vi "AlliGator Get HDF5 File Type.vi"(8 "Error In":errorcluster, 11 "File Path":path) -> (0 "Error Out":errorcluster, 3 "File Type":string)   [LabVIEW 2021, in "AlliGator HDF5.lvlib"]
uses:
  AlliGator HDF5.lvlib
  <vilib>/addons/h5labview2/base/hid_t.ctl
  <vilib>/addons/h5labview2/base/H5Equery.vi
  <vilib>/addons/h5labview2/base/lib_path.vi
  <vilib>/addons/h5labview2/dataset/H5Dread.llb/H5Dread.xnode
  <vilib>/addons/h5labview2/group/H5G.lvlib
  <vilib>/addons/h5labview2/file/H5F.lvlib
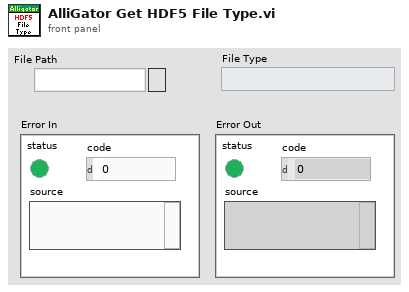
[diagram p1: front panel]
types:
  T1 = typedef "hid_t.ctl" = i64
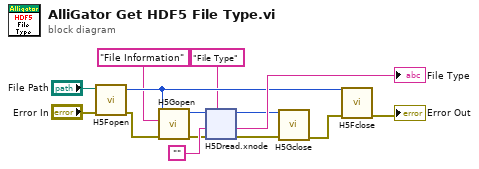
[diagram p0: block diagram]
diagram:
  n1 = call <vilib>:"H5Fopen.vi"("error in (no error)"="Error In", "path"="File Path") -> ("error out"=w3:errorcluster, "ref out"=w12:T1)  [unwired: 8 in]
  n2 = call <vilib>:"H5Gopen.vi"("error in (no error)"=w3, "name"="File Information" ("dataset name (this)"), "ref in"=w12) -> ("error out"=w5:errorcluster, "group out"=w6:T1)  [unwired: 7 in]
  n3 = xnode "H5Dread.xnode"("dataset name (this)"="File Type", "error in (no error)"=w5, "default"="", "ref in"=w6) -> ("error out"=w9:errorcluster, "data"=→"File Type":string, "ref out"=w8:T1)  [unwired: 2 in, 1 out]
  n4 = call <vilib>:"H5Gclose.vi"("error in (no error)"=w9, "group in"=w8) -> ("error out"=w11:errorcluster)  [unwired: 9 in]
  n5 = call <vilib>:"H5Fclose.vi"("error in (no error)"=w11, "ref"=w12) -> ("error out"=→"Error Out":errorcluster)  [unwired: 9 in]
